vi "proptest_runtime class.vi"() -> ()   [LabVIEW 2013, in "TBM Tests.lvlib"]
uses:
  TBM Tests.lvlib
  root configuration/TBM configuration.lvclass
panel:
  out "error 538305":errorcluster
  out "class name empty=ok":bool
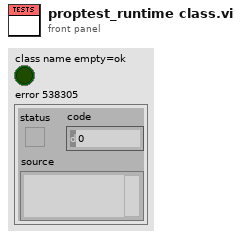
[diagram p1: front panel]
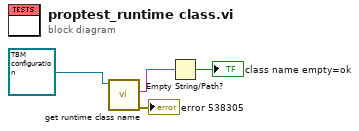
[diagram p0: block diagram]
diagram:
  n1 = call-dynamic "get runtime class name.vi"("configuration in"=refnum<class "TBM configuration.lvclass"> refnum ("configuration")) -> ("error out"=→"error 538305":errorcluster, "class name"=w3:string)  [unwired: 8 in, 1 out]
  n2 = Empty String/Path?(string/path=w3) -> (empty?=→"class name empty=ok":bool)
